vi "FindTurnDistanceCamreon.vi"(8 "Current":dbl, 11 "Wanted":dbl) -> (1 "Negate":bool, 2 "Distance":dbl)   [LabVIEW 2017]
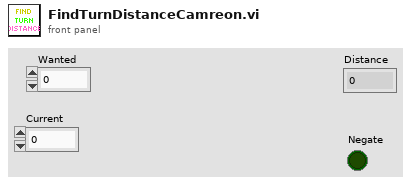
[diagram p1: front panel]
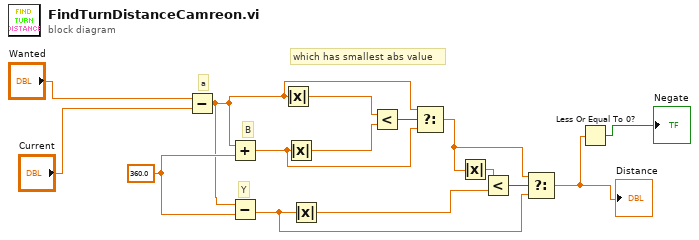
[diagram p0: block diagram]
diagram:
  w13 = 360.0
  # "which has smallest abs value"
  # "Y"
  # "B"
  # "a"
  n1 = Subtract(x="Wanted", y="Current") -> (x-y=w9:dbl)
  n2 = Add(x=w9, y=w13) -> (x+y=w8:dbl)
  n3 = Subtract(x=w9, y=w13) -> (x-y=w3:dbl)
  n4 = Absolute Value(x=w9) -> (abs(x)=w11:dbl)
  n5 = Absolute Value(x=w8) -> (abs(x)=w10:dbl)
  n6 = Absolute Value(x=w3) -> (abs(x)=w6:dbl)
  n7 = Less?(x=w11, y=w10) -> (x < y?=w12:bool)
  n8 = Select(t=w9, s=w12, f=w8) -> (s? t:f=w4:dbl)
  n9 = Absolute Value(x=w4) -> (abs(x)=w5:dbl)
  n10 = Less?(x=w5, y=w6) -> (x < y?=w7:bool)
  n11 = Select(t=w4, s=w7, f=w3) -> (s? t:f=w2:dbl)
  "Distance" <- w2
  n12 = Less Or Equal To 0?(x=w2) -> (x <= 0?=→"Negate":bool)
